vi "parse unique name.vi"(11 "unique ring name":string) -> (2 "UID":string, 3 "alias":string)   [LabVIEW 2013, in "PL Framework Configuration Tool.lvlib" / "Engine Mappings.lvclass"]
uses:
  Engine Mappings.lvclass
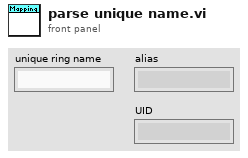
[diagram p1: front panel]
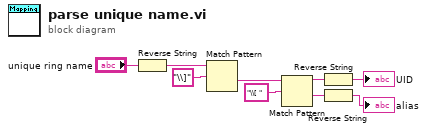
[diagram p0: block diagram]
diagram:
  n1 = Reverse String(1:"unique ring name") -> (0:w8:string)
  n2 = Match Pattern(string=w8, regular expression="\\]") -> (after substring=w6:string)  [unwired: 1 in, 3 out]
  n3 = Match Pattern(string=w6, regular expression="\\[ " ("string")) -> (before substring=w5:string, after substring=w4:string)  [unwired: 1 in, 2 out]
  n4 = Reverse String(1:w5) -> (0:→"UID":string)
  n5 = Reverse String(1:w4) -> (0:→"alias":string)
